vi "OxITC503 _Query_ Version.vi"(0 "VISA session":refnum<visa-resource-name>, 1 "error in":errorcluster) -> (2 "VISA session":refnum<visa-resource-name>, 3 "Version String":string, 4 "error out (no error)":errorcluster)   [LabVIEW 2013]
doc: "Returns a message indicating the instrument type and the firmware version number."
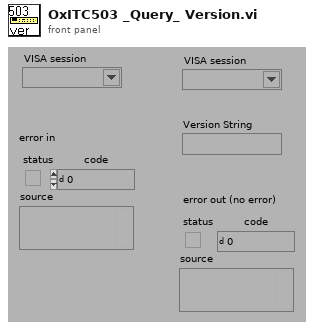
[diagram p1: front panel]
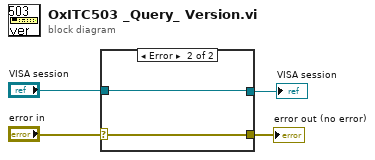
[diagram p0: block diagram]
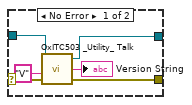
[diagram p2: hidden frame]
diagram:
  n1 = case shown="Error" "error in" {
    selector: "error in" -> [w5 w11]
    tunnel: [w9 w11] -> w4
    tunnel: "VISA session" -> [w7 w12]
    tunnel: [w6 w12] -> w2
    frame No Error {
      n2 = call "OxITC503 _Utility_ Talk.vi"("VISA session"=w7, "Command"="V", "error in (no error)"=w5) -> ("VISA session"=w6:refnum<visa-resource-name>, "read buffer"=→"Version String":string, "error out (no error)"=w9:errorcluster)  [unwired: 2 in]
    }
    frame Error {
    }
  }
  "error out (no error)" <- w4
  "VISA session" <- w2
